vi "mean_result.vi"(7 "FGV_mods":T1, 8 "Error In":errorcluster, 11 "inert":waveform(dbl)[](array[waveform])) -> (0 "Error Out":errorcluster)   [LabVIEW 2017]
uses:
  mean_result_mods.ctl
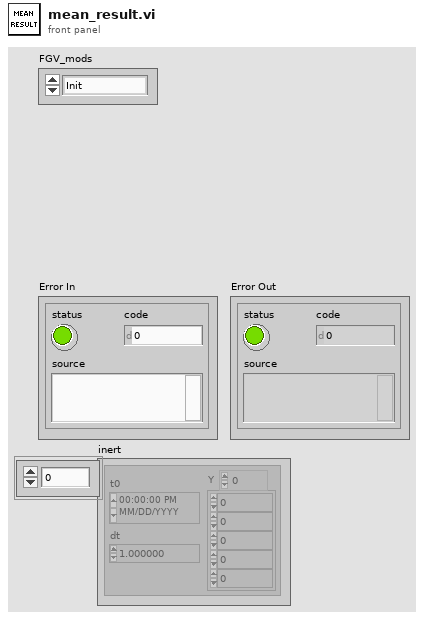
[diagram p1: front panel]
types:
  T1 = typedef "mean_result_mods.ctl" = enum16{"Init", "Clear", "NewHit"}
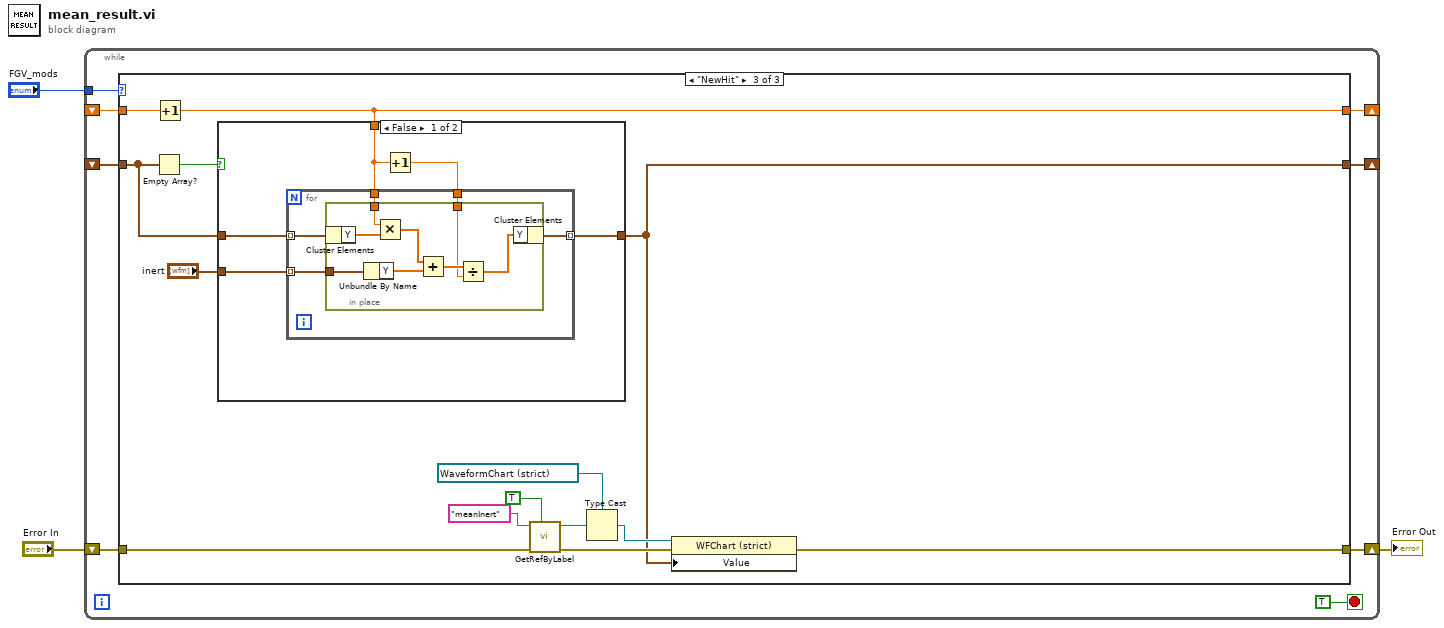
[diagram p0: block diagram]
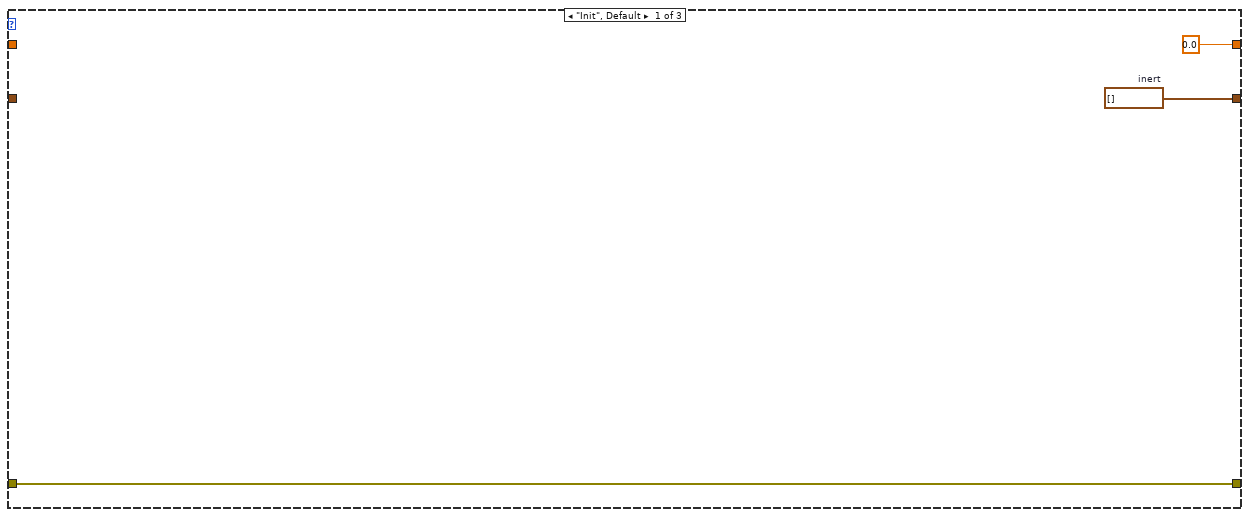
[diagram p2: hidden frame]
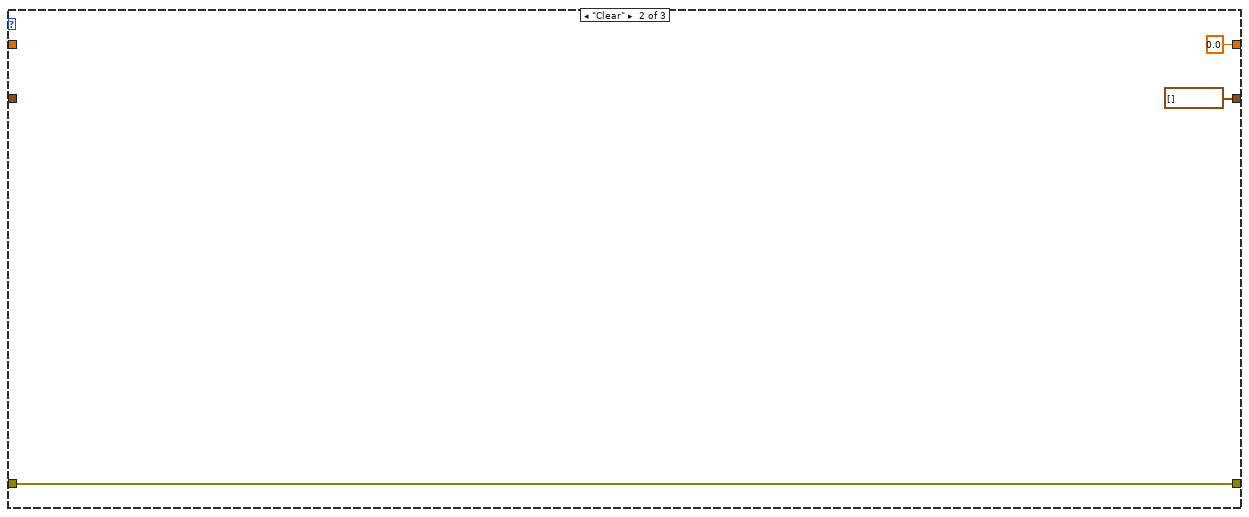
[diagram p3: hidden frame]
diagram:
  n1 = while {
    tunnel: "FGV_mods" -> [w10]
    shift-right: [w9] -> _
    shift-left: _ -> [w8]
    shift-right: [w6] -> w1
    shift-left: "Error In" -> [w7]
    shift-right: [w5] -> _
    shift-left: _ -> [w4]
    stop <- TRUE stop-if-true
    n2 = case shown="\"NewHit\"" w10 {
      tunnel: [w13 waveform(dbl)[] [] ("inert") w19] -> w9
      tunnel: w8 -> [_ _ w28]
      tunnel: w7 -> [w14 w17 w20]
      tunnel: [w14 w17 w18] -> w6
      tunnel: [0.0 0.0 w27] -> w5
      tunnel: w4 -> [_ _ w29]
      frame "Init", Default {
        w13 = waveform(dbl)[] []  # inert
      }
      frame "Clear" {
      }
      frame "NewHit" {
        n3 = Empty Array?(array=w28) -> (empty?=w31:bool)
        n4 = Increment(x=w29) -> (x+1=w27:dbl)
        n5 = case shown="False" w31 {
          tunnel: [w32 w50] -> w19
          tunnel: "inert" -> [w35 w50]
          tunnel: w28 -> [w36 _]
          tunnel: w27 -> [w34 _]
          frame False {
            n6 = Increment(x=w34) -> (x+1=w33:dbl)
            n7 = for {
              tunnel: w36 -> [w41] mode=indexing
              tunnel: w35 -> [w40] mode=indexing
              tunnel: w34 -> [w39]
              tunnel: w33 -> [w38]
              tunnel: [w37] -> w32 mode=indexing
              n8 = in-place {
                in-place-border: w39 -> [w48]
                in-place-border: w40 -> [w46]
                in-place-border: w38 -> [w43]
                n9 = in-place-cluster #1(w41) -> ("Y"=w49:dbl[])
                n10 = Unbundle By Name(w46) -> ("Y"=w45:dbl[])
                n11 = Multiply(x=w48, y=w49) -> (x*y=w47:dbl[])
                n12 = Add(x=w47, y=w45) -> (x+y=w44:dbl[])
                n13 = Divide(x=w44, y=w43) -> (x/y=w42:dbl[])
                n14 = in-place-cluster #1("Y"=w42) -> (w37:waveform(dbl))
              }
            }
          }
          frame True {
          }
        }
        n15 = call "GetRefByLabel.vi"("InsideTab"=TRUE, "error in"=w20, "Label"="meanInert") -> ("error out"=w25:errorcluster, "Ctl Refnum"=w24:refnum<vi>)  [unwired: 6 in, 1 out]
        n16 = Type Cast(type=refnum<vi> refnum ("acelTime"), x=w24) -> (*(type *) &x=w26:refnum<vi>)
        n17 = property class="WFChart (strict)"(reference=w26, error in=w25, "Value"=w19) -> (error out=w18:errorcluster)  [unwired: 1 out]
      }
    }
  }
  "Error Out" <- w1
